vi "PointToSetting.vi"(10 "Clicked":dbl[](array[numeric]), 11 "Scan Settings":T1={"XStart"=-200000000, "XEnd"=200000000, "XNum"=500, "YStart"=-200000000, "YEnd"=200000000, "YNum"=500, "ZStart"=0, "ZEnd"=0, "ZNum"=1}) -> (3 "Setting":i32[](array[numeric]))   [LabVIEW 2012]
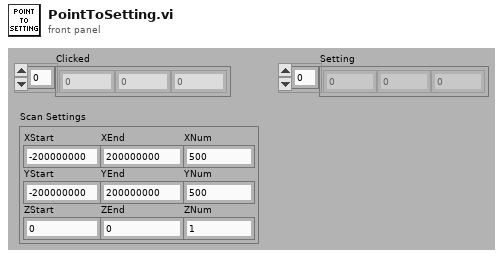
[diagram p1: front panel]
types:
  T1 = cluster{"XStart":i32, "XEnd":i32, "XNum":i32, "YStart":i32, "YEnd":i32, "YNum":i32, "ZStart":i32, "ZEnd":i32, "ZNum":i32}
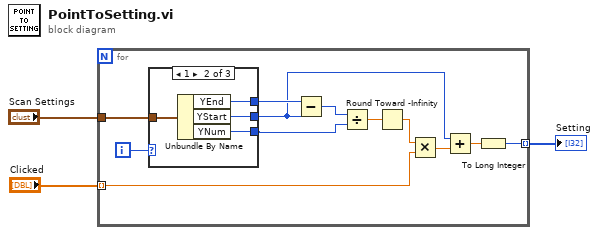
[diagram p0: block diagram]
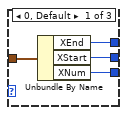
[diagram p2: hidden frame]
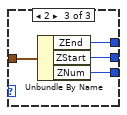
[diagram p3: hidden frame]
diagram:
  n1 = for {
    tunnel: "Clicked" -> [w8] mode=indexing
    tunnel: "Scan Settings" -> [w15]
    tunnel: [w4] -> w1 mode=indexing
    i -> [w14]
    n2 = case shown="1" w14 {
      tunnel: w15 -> [w19 w23 w27]
      tunnel: [w18 w22 w26] -> w9
      tunnel: [w17 w21 w25] -> w6
      tunnel: [w16 w20 w24] -> w10
      frame 0, Default {
        n3 = Unbundle By Name(w19) -> ("XEnd"=w18:i32, "XStart"=w17:i32, "XNum"=w16:i32)
      }
      frame 1 {
        n4 = Unbundle By Name(w23) -> ("YEnd"=w22:i32, "YStart"=w21:i32, "YNum"=w20:i32)
      }
      frame 2 {
        n5 = Unbundle By Name(w27) -> ("ZEnd"=w26:i32, "ZStart"=w25:i32, "ZNum"=w24:i32)
      }
    }
    n6 = Subtract(x=w9, y=w6) -> (x-y=w11:i32)
    n7 = Divide(x=w11, y=w10) -> (x/y=w12:dbl)
    n8 = Round Toward -Infinity(1:w12) -> (0:w13:dbl)
    n9 = Multiply(x=w13, y=w8) -> (x*y=w7:dbl)
    n10 = Add(x=w6, y=w7) -> (x+y=w5:dbl)
    n11 = To Long Integer(number=w5) -> (32bit integer=w4:i32)
  }
  "Setting" <- w1
